vi "Calibration Audit v2.vi"() -> ()   [LabVIEW 2014]
doc: "Obtains calibration information for hardware on selected target."
uses:
  <vilib>/nisyscfg/nisyscfg.lvlib
  <resource>/objmgr/nisysapi.rc
  <vilib>/Utility/miscctls.llb/LVRowAndColumnTypeDef.ctl
  <vilib>/Utility/error.llb/DialogType.ctl
  States.ctl
  <vilib>/Utility/sysdir.llb/System Directory Type.ctl
  <vilib>/Utility/file.llb/Write To Spreadsheet File (string).vi
  <vilib>/nisyscfg/Close (Hardware).vi
  <vilib>/nisyscfg/Close (System).vi
  <vilib>/nisyscfg/Close (Filter).vi
panel:
  in  "Discover Remote Devices?":bool
  in  "Stop Button":bool
  out "Display":string
  in  "User Inputs":T1={"Target "="localhost", "User Name"="", "Password "="", "Filter Enabled?"=FALSE, "Cal File Destination"=path ""}
  in  "START":bool
  out "Calibration Results":string[][](table)
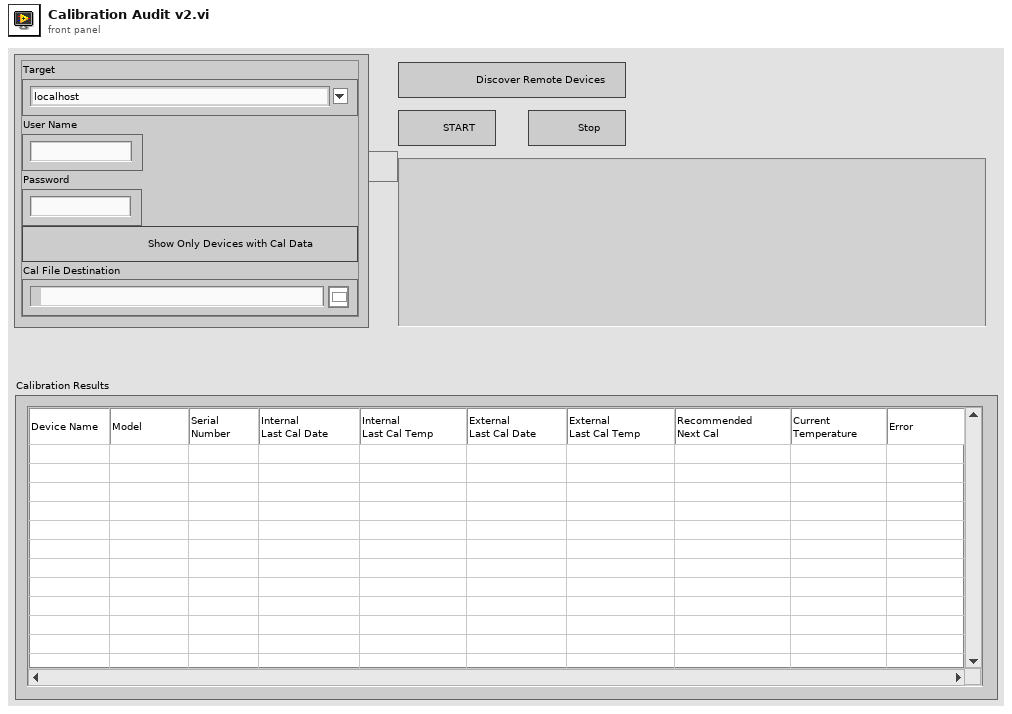
[diagram p1: front panel]
types:
  T1 = cluster{"Target ":string, "User Name":string, "Password ":string, "Filter Enabled?":bool, "Cal File Destination":path}
  T2 = cluster{"SysConfig Session":refnum<k21>, "SysConfig Filter":refnum<k20>, "Modules to Cal":refnum<k20>[], "Cal Data to Write":string[][], "ComboBox Values":string[]}
  T3 = typedef "States.ctl" = enum16{"Initialize", "List Known Systems", "Discover Remote", "Wait for Event", "Filter and Validate", "Update Cal Data", "Report Cal Data", "Close"}
  T4 = cluster{"User Inputs":cluster{"Target ":string, "User Name":string, "Password ":string, "Filter Enabled?":bool, "Cal File Destination":path}, "Display":refnum<vi>, "Target ":refnum<vi>}
  T5 = typedef "LVRowAndColumnTypeDef.ctl" = cluster{"Row":i32, "Column":i32}
  T6 = typedef "System Directory Type.ctl" = i32
  T7 = typedef "DialogType.ctl" = u16
  T8 = cluster{"Last Calibrated":timestamp, "Last Temperature":dbl, "Recommended Next Calibration":timestamp}
  T9 = cluster{"Last Calibrated":timestamp, "Last Temperature":dbl}
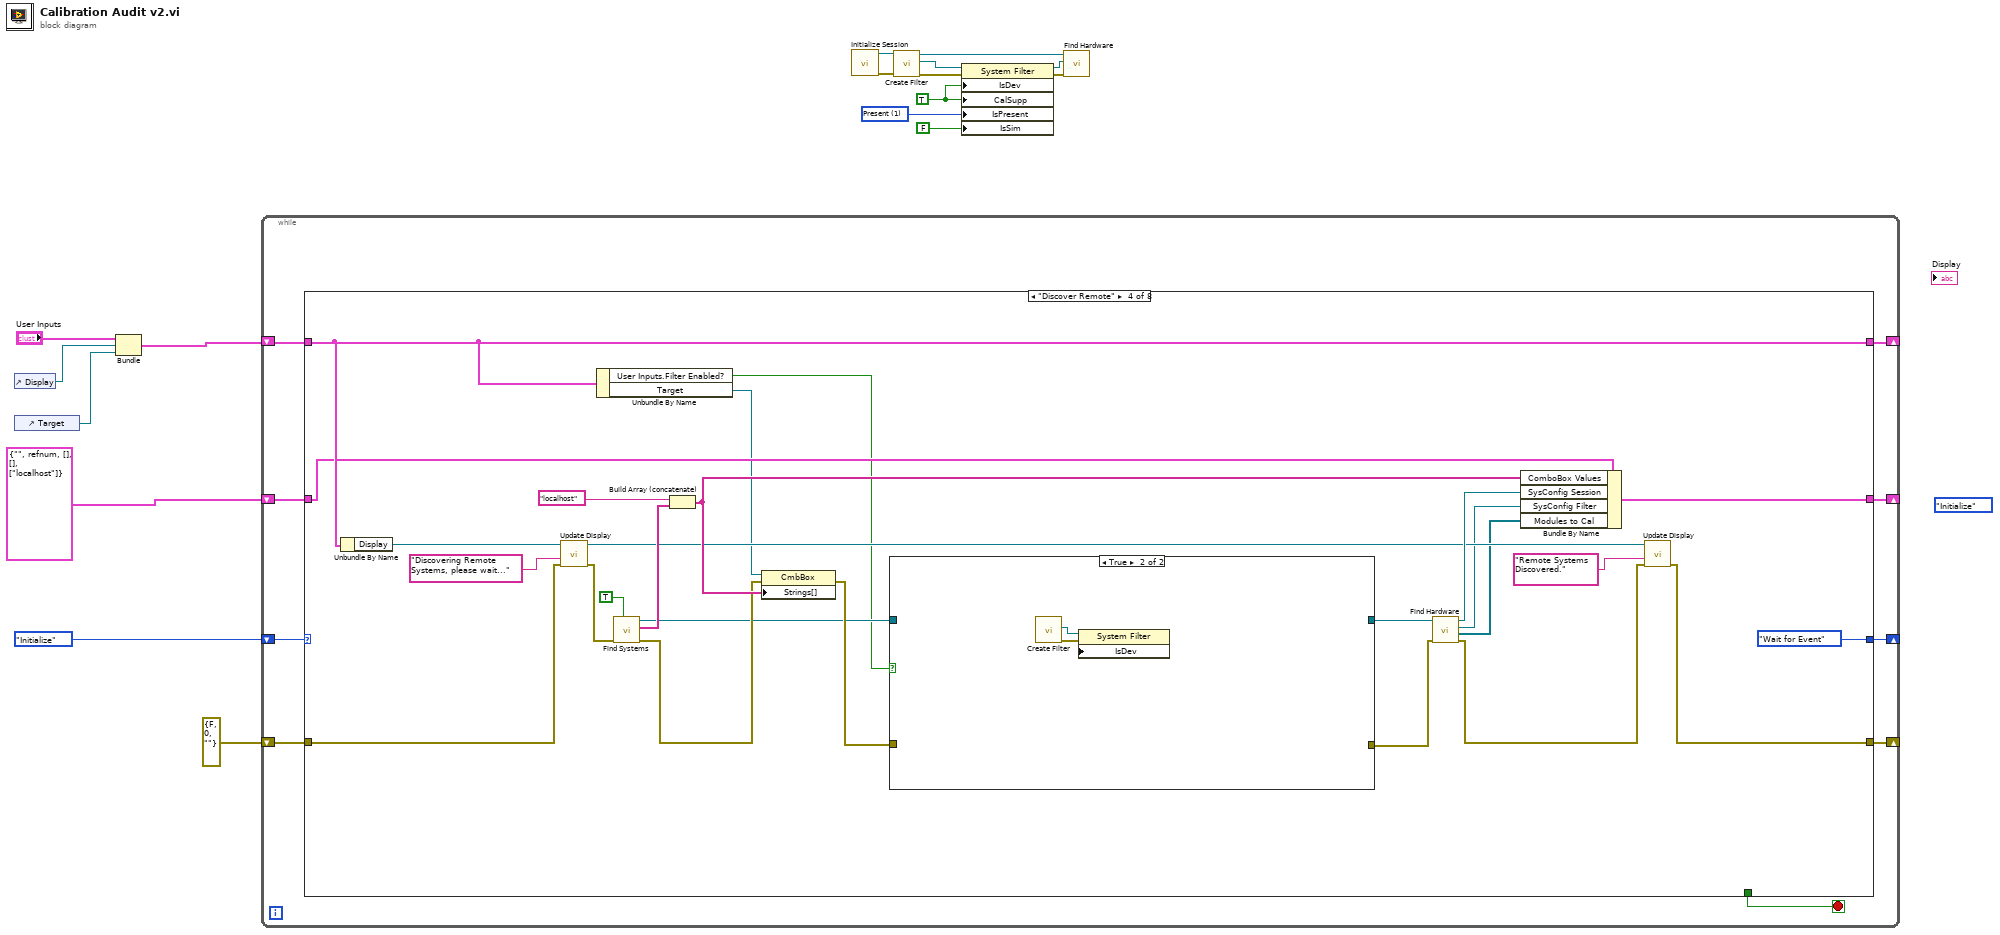
[diagram p0: block diagram]
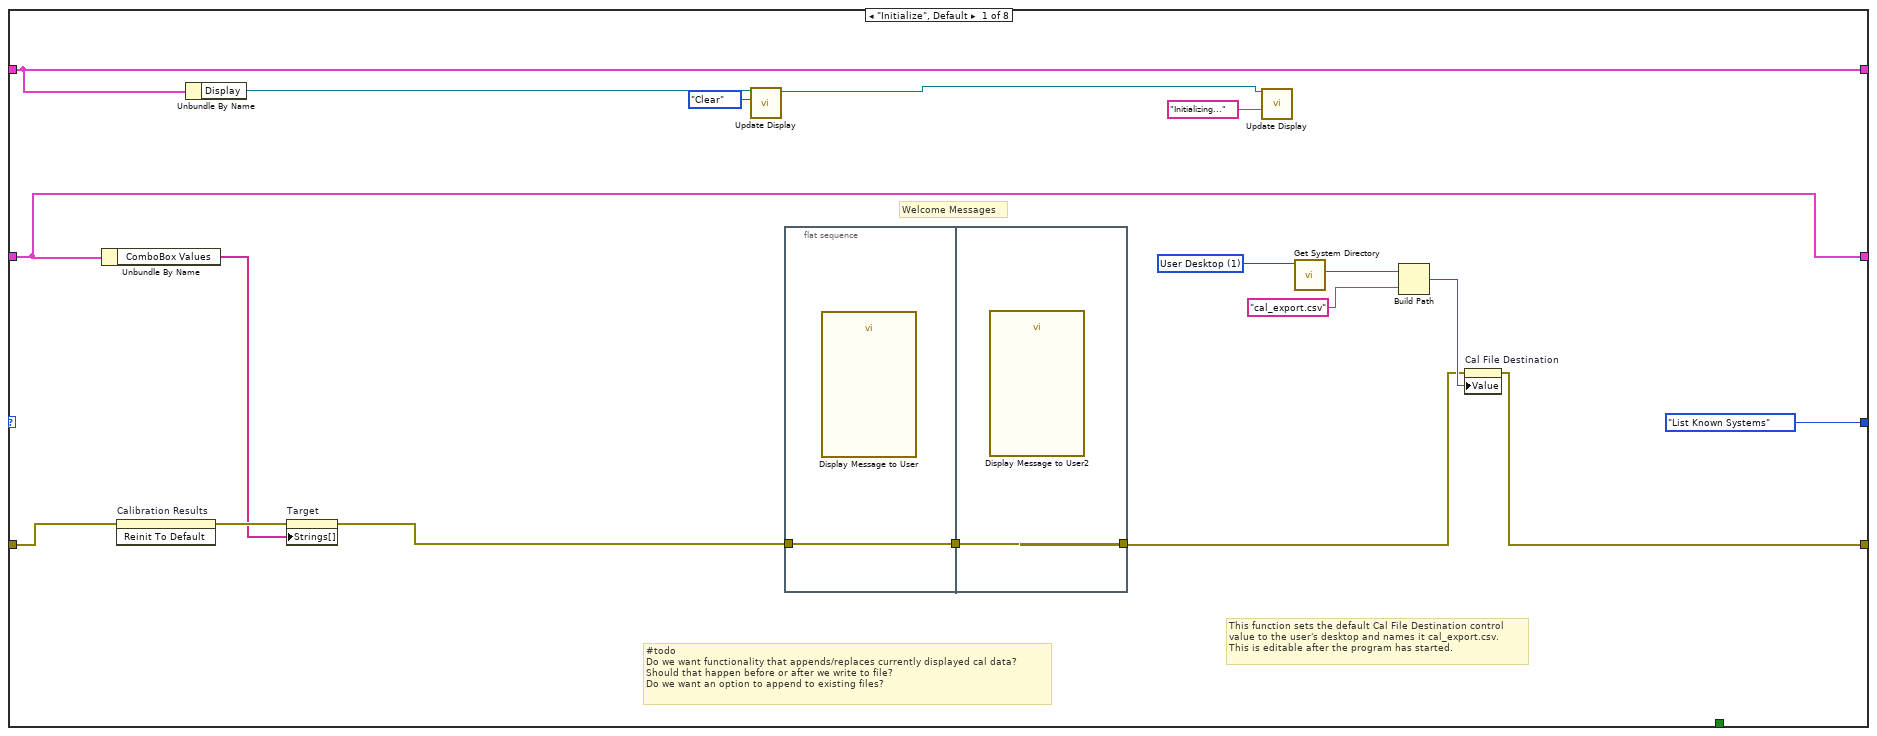
[diagram p2: hidden frame]
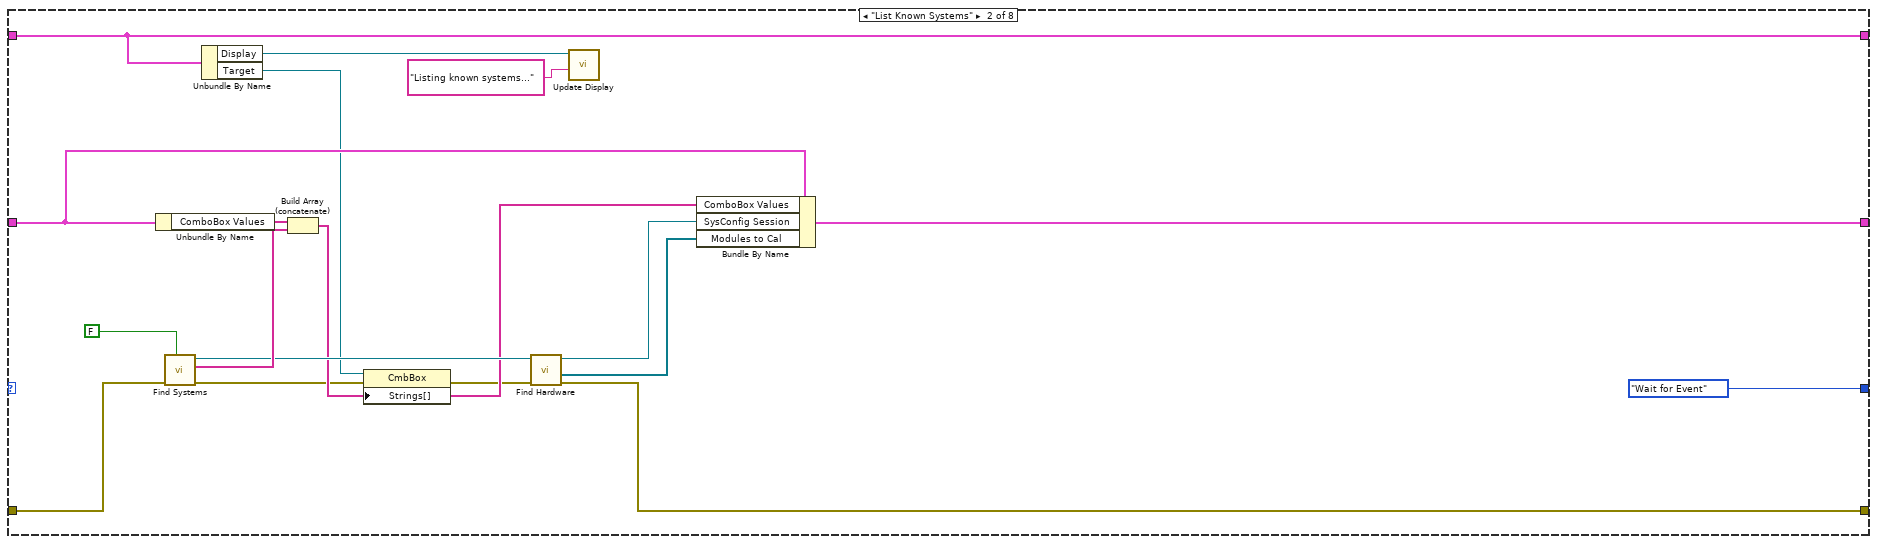
[diagram p3: hidden frame]
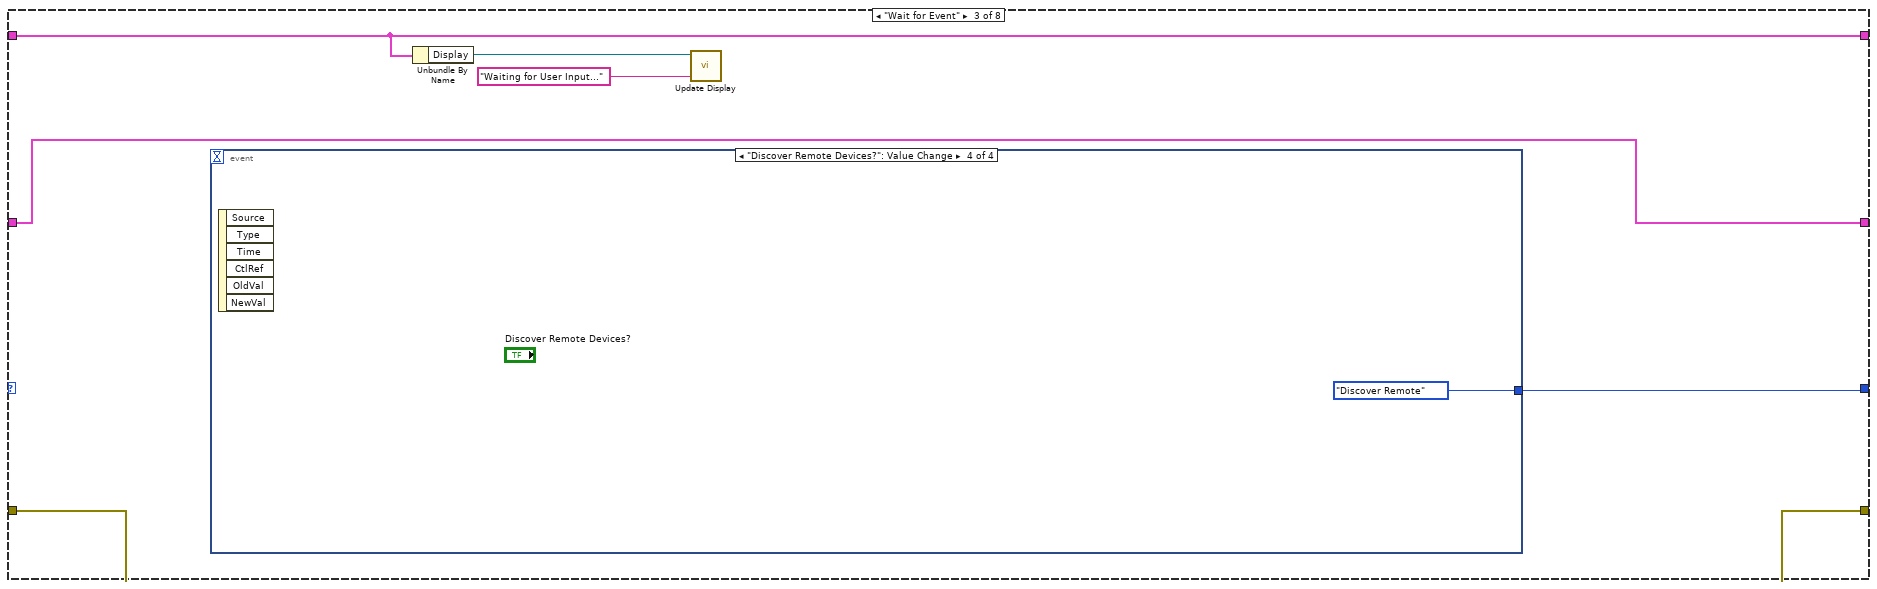
[diagram p4: hidden frame]
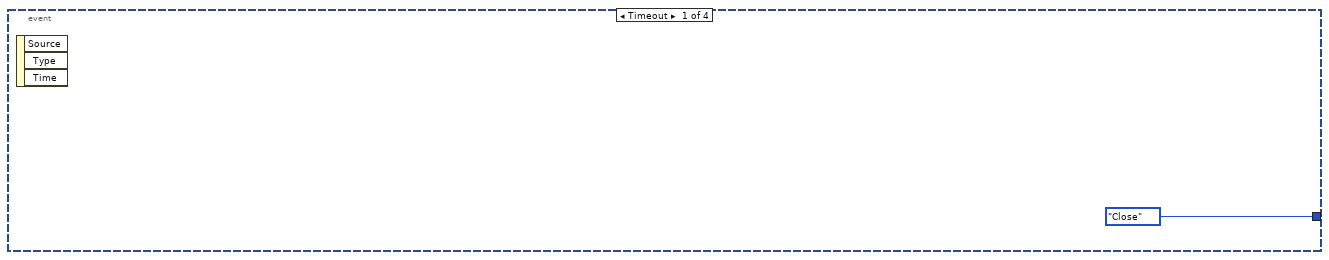
[diagram p5: hidden frame]
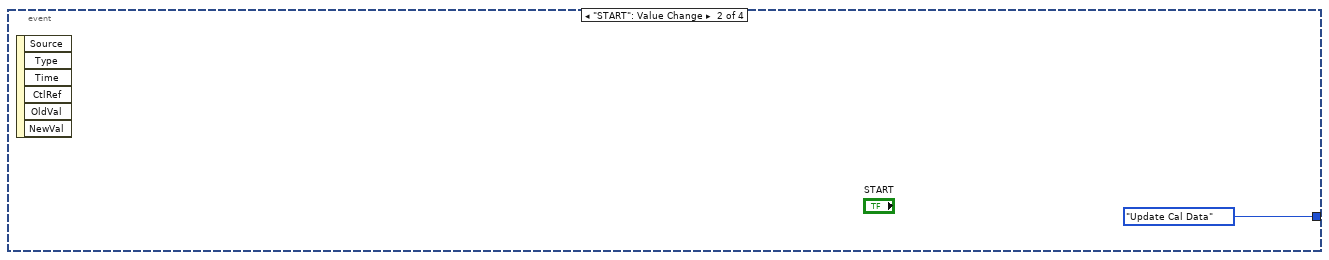
[diagram p6: hidden frame]
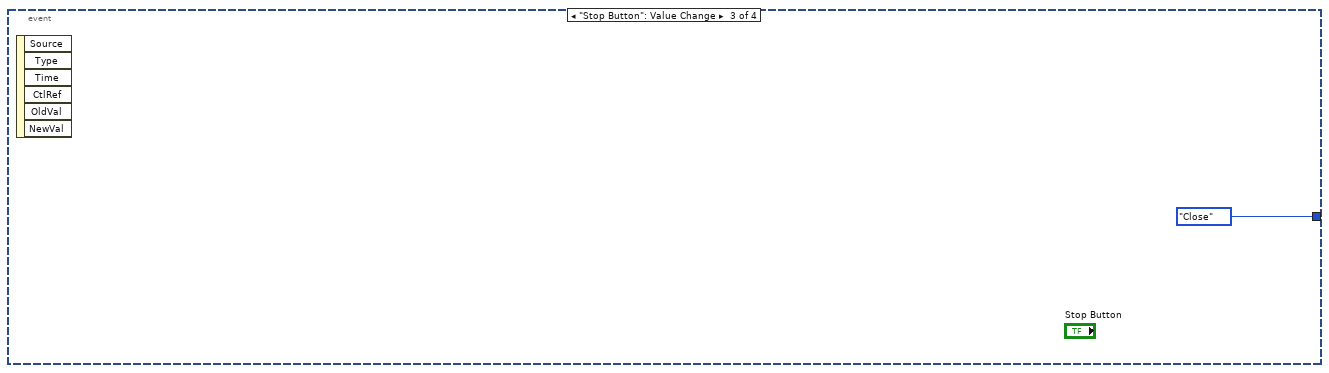
[diagram p7: hidden frame]
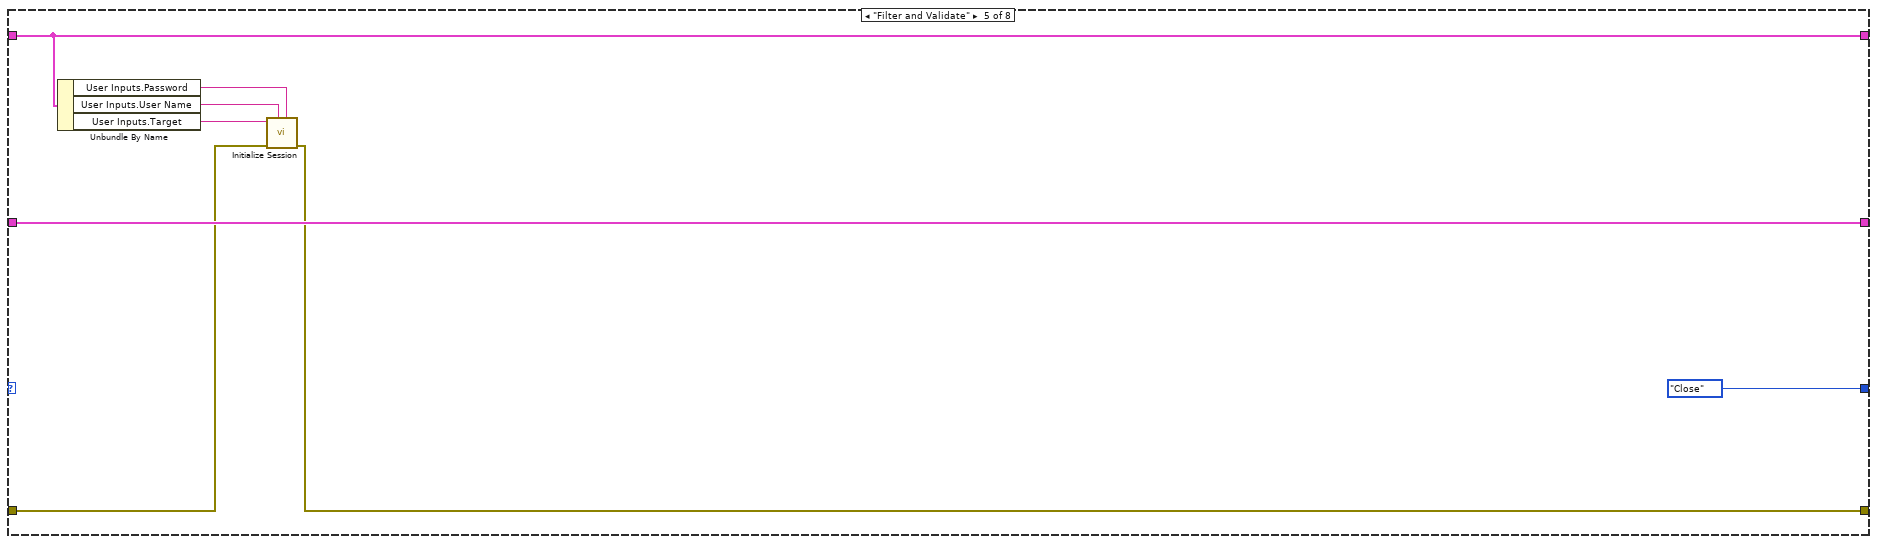
[diagram p9: hidden frame]
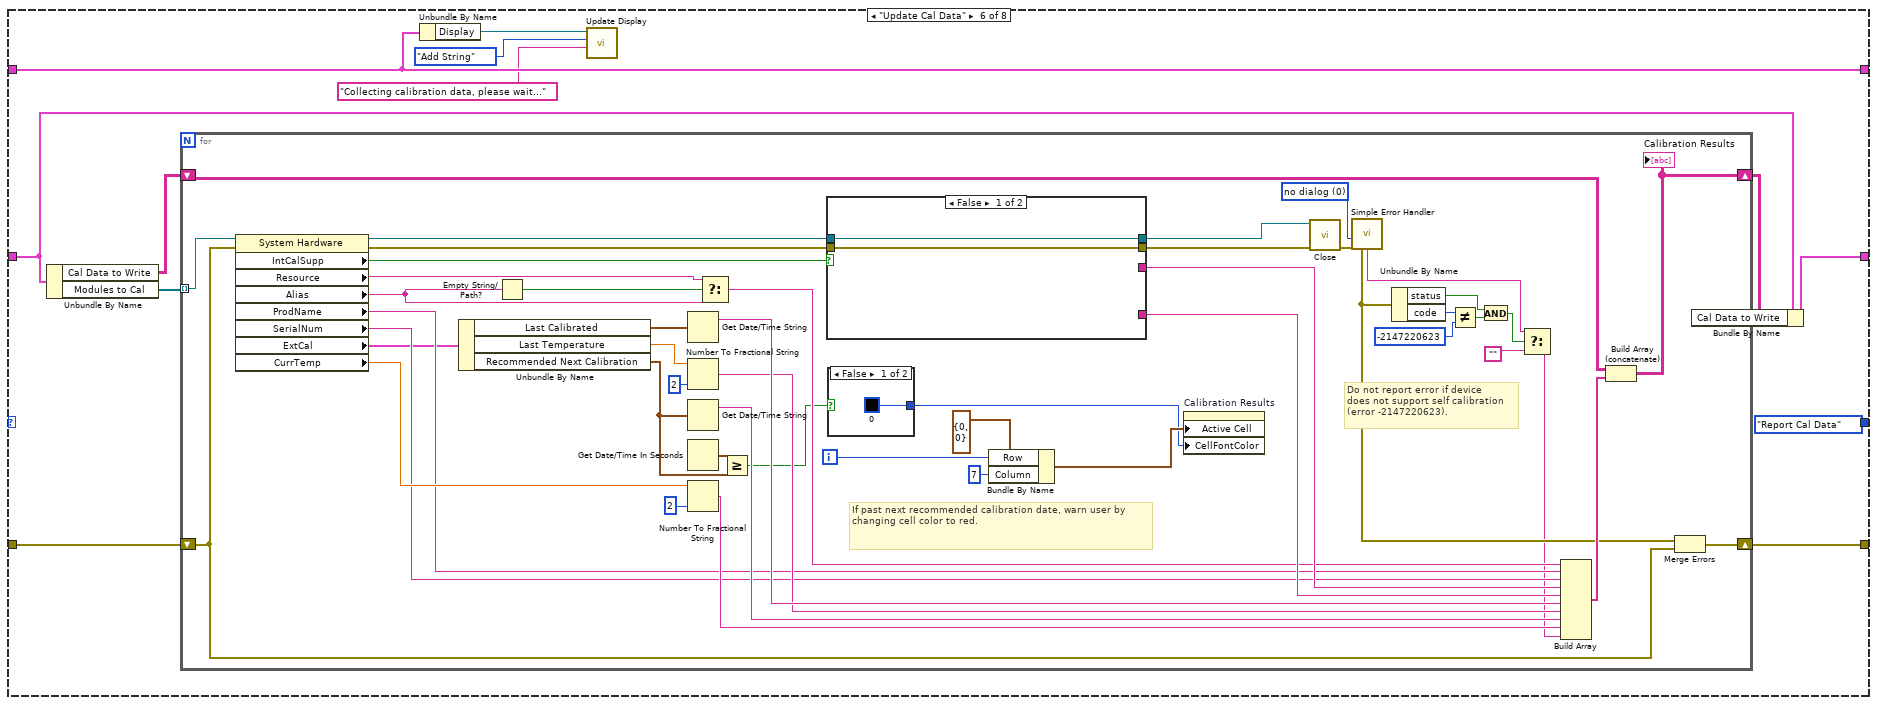
[diagram p10: hidden frame]
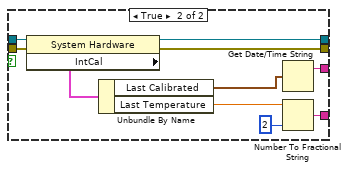
[diagram p11: hidden frame]
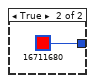
[diagram p12: hidden frame]
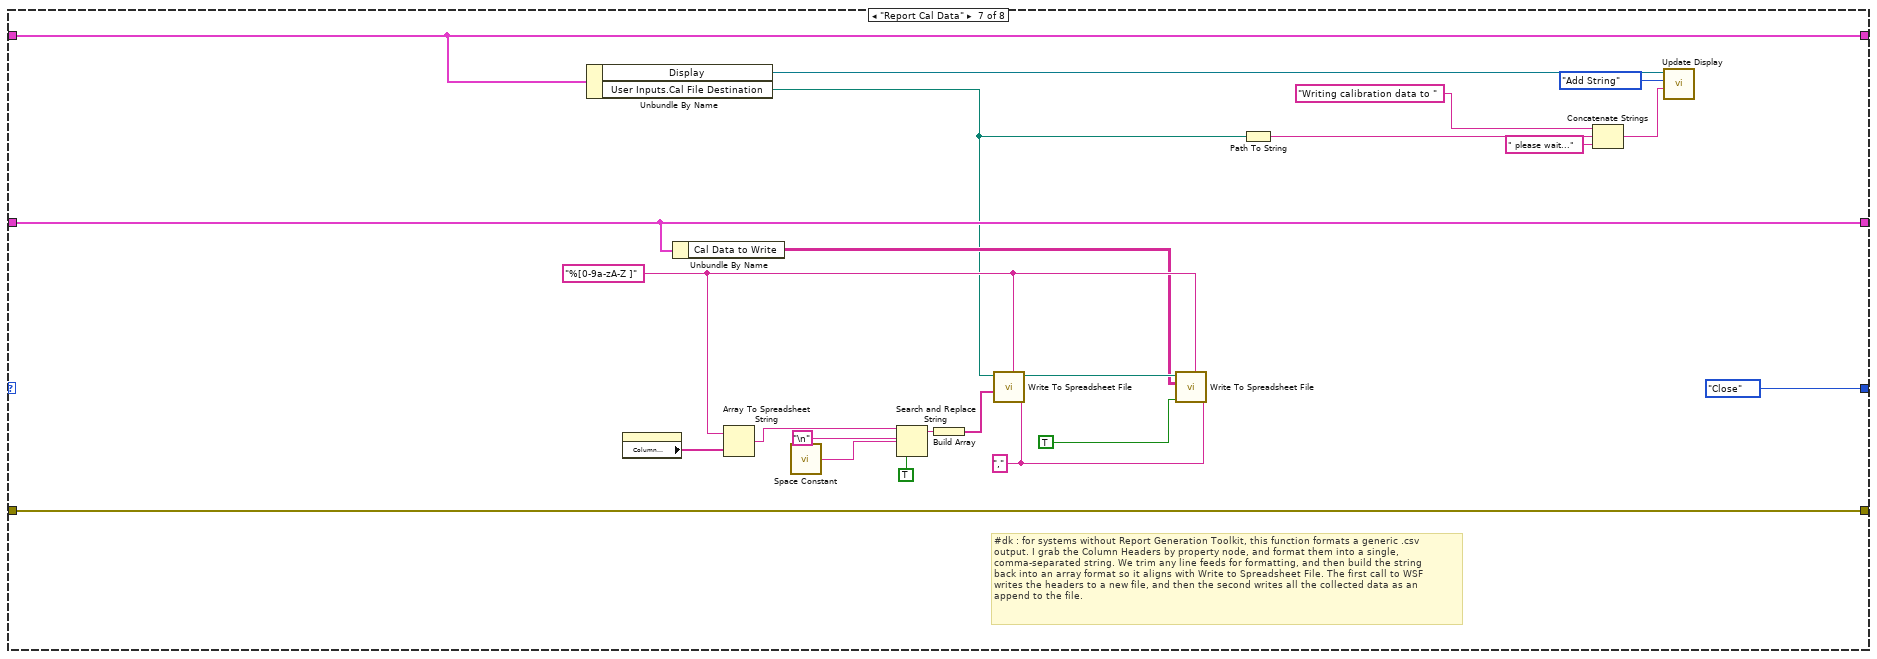
[diagram p13: hidden frame]
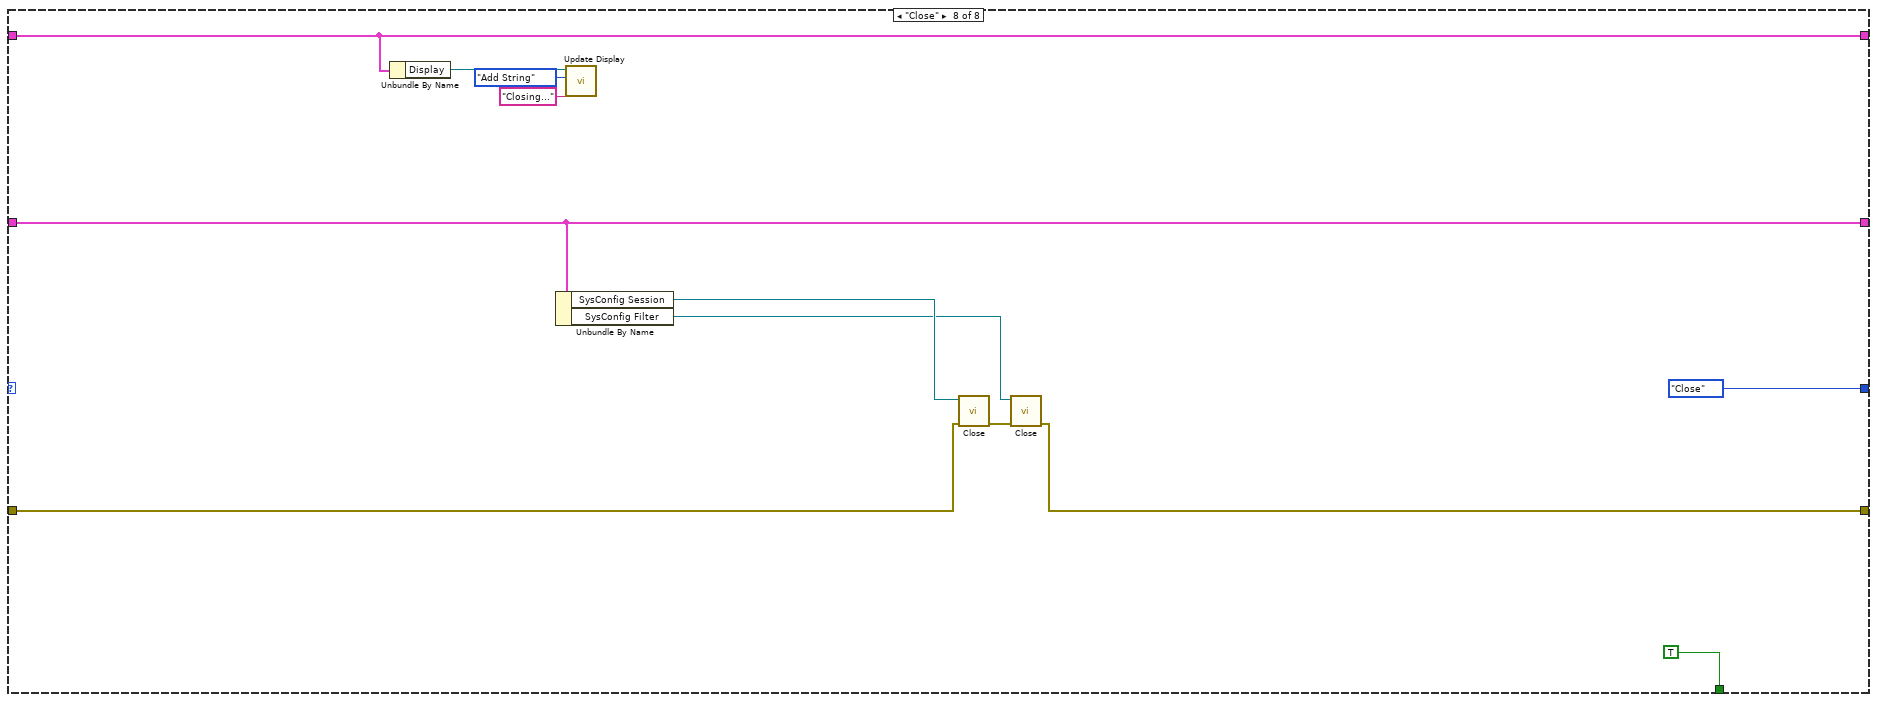
[diagram p14: hidden frame]
diagram:
  (unwired) States."Initialize"
  w13 = 1 items=["Unknown"=-1, "Not Present"=0, "Present"=1] ("Is Present")
  w9 = TRUE ("Is Device")
  n1 = control-ref of="Display"() -> (w2:refnum<vi>)
  n2 = control-ref of="Target"() -> (w1:refnum<vi>)
  n3 = Bundle("User Inputs"="User Inputs", "Display"=w2, "Target"=w1) -> (w5:T4)  [unwired: 1 in]
  n4 = while {
    shift-right: [w22] -> _
    shift-left: States."Initialize" -> [w18]
    shift-right: [w23] -> _
    shift-left: errorcluster {"status"=FALSE, "code"=0, "source"=""} ("error constant") -> [w26]
    shift-right: [w24] -> _
    shift-left: w5 -> [w25]
    shift-right: [w20] -> _
    shift-left: T2 {"SysConfig Session"="", "SysConfig Filter"=refnum, "Modules to Cal"=[], "Cal Data to Write"=[], "ComboBox Values"=["localhost"]} -> [w19]
    stop <- w21 stop-if-true
    n5 = case shown="\"Discover Remote\"" w18 {
      tunnel: w26 -> [w32 w57 w70 w90 w107 w123 w197 w215]
      tunnel: w25 -> [w36 w62 w67 w92 w111 w116 w195 w212]
      tunnel: [w36 w62 w67 w92 w111 w116 w195 w212] -> w24
      tunnel: [w38 w54 w70 w86 w105 w122 w197 w214] -> w23
      tunnel: [States."List Known Systems" States."Wait for Event" w69 States."Wait for Event" States."Close" States."Report Cal Data" States."Close" States."Close"] -> w22
      tunnel: [_ _ _ _ _ _ _ TRUE] -> w21
      tunnel: [w29 w63 w68 w89 w112 w117 w194 w217] -> w20
      tunnel: w19 -> [w29 w59 w68 w84 w112 w118 w194 w217]
      frame "Initialize", Default {
        w44 = T6 1 items=["User Home"=0, "User Desktop"=1, "User Documents"=2, "User Application Data"=3, "User Preferences"=4, "User Temporary"=5, "Public Documents"=6, "Public Application Data"=7, "Public Preferences"=8, "Public Cache"=13, "System Core Libraries"=9, "System Installed Libraries"=10, "Application Files"=11, "Boot Volume Root"=12] ("system directory type")
        # "#todo \nDo we want functionality that appends/replaces currently displayed cal data?\nShould that happen before or after we write to file? \nDo we want an option to append to existing files?"
        # "Welcome Messages"
        # "This function sets the default Cal File Destination control\nvalue to the user's desktop and names it cal_export.csv. \nThis is editable after the program has started."
        n6 = Unbundle By Name(w29) -> ("ComboBox Values"=w28:string[])
        n7 = invoke on="Calibration Results" class="Tbl (strict)" method="Reinit To Default"(error in=w32) -> (error out=w31:errorcluster)  [unwired: 2 in, 2 out]
        n8 = Unbundle By Name(w36) -> ("Display"=w35:refnum<vi>)
        n9 = property on="Target" class="CmbBox"(error in=w31, "Strings[]"=w28) -> (error out=w30:errorcluster)  [unwired: 1 in, 1 out]
        n10 = call "Update Display.vi"("Action"=enum16{"Add String", "Newline", "Clear"}."Clear", "Display In"=w35) -> ("Display Out"=w34:refnum<vi>)  [unwired: 8 in, 1 out]
        n11 = flat-sequence {
          tunnel: w30 -> [w45]
          tunnel: [w45] -> w41
          tunnel: [w46] -> w39
          tunnel: w41 -> [w46]
          frame #0 {
            n12 = call "Display Message to User"() -> ()  [unwired: 10 in, 2 out]
          }
          frame #1 {
            n13 = call "Display Message to User2"() -> ()  [unwired: 10 in, 2 out]
          }
        }
        n14 = call "Update Display.vi"("string"="Initializing...", "Display In"=w34) -> ()  [unwired: 8 in, 2 out]
        n15 = call <vilib>:"Get System Directory.vi"("system directory type"=w44) -> ("system directory"=w42:path)  [unwired: 10 in]
        n16 = Build Path(base path=w42, name or relative path="cal_export.csv") -> (appended path=w40:path)
        n17 = property on="Cal File Destination" class="Path"(error in=w39, "Value"=w40) -> (error out=w38:errorcluster)  [unwired: 1 in, 1 out]
      }
      frame "List Known Systems" {
        n18 = Unbundle By Name(w59) -> ("ComboBox Values"=w56:string[])
        n19 = call <vilib>:"Find Systems.vi"("Detect Online Systems (T)"=FALSE, "error in (no error)"=w57) -> ("error out"=w49:errorcluster, "Detected Systems"=w58:string[], "Session out"=w55:refnum<k21>)  [unwired: 7 in]
        n20 = Unbundle By Name(w62) -> ("Display"=w61:refnum<vi>, "Target"=w51:refnum<vi>)
        n21 = Build Array (concatenate)(w56, w58) -> (w50:string[])
        n22 = property class="CmbBox"(reference=w51, error in=w49, "Strings[]"=w50) -> (error out=w48:errorcluster)  [unwired: 1 out]
        n23 = call <vilib>:"Find Hardware.vi"("error in (no error)"=w48, "Session in"=w55) -> ("error out"=w54:errorcluster, "Resources out"=w52:refnum<k20>[], "Session out"=w53:refnum<k21>)  [unwired: 6 in, 1 out]
        n24 = call "Update Display.vi"("string"="Listing known systems...", "Display In"=w61) -> ()  [unwired: 8 in, 2 out]
        n25 = Bundle By Name(cluster=w59, "ComboBox Values"=w50, "SysConfig Session"=w53, "Modules to Cal"=w52) -> (w63:T2)
      }
      frame "Wait for Event" {
        n26 = event shown="[3] \"Discover Remote Devices?\": Value Change" {
          selector: _ -> [_ _ _ _]
          dyn-events: _ -> [_ _ _ _]
          timeout: _ -> [_ _ _ _]
          tunnel: [States."Close" States."Update Cal Data" States."Close" States."Discover Remote"] -> w69
          event Timeout {
            n27 = event-data() -> ()  [unwired: 1 in, 3 out]
          }
          event "START": Value Change {
            n28 = event-data() -> ()  [unwired: 1 in, 6 out]
          }
          event "Stop Button": Value Change {
            n29 = event-data() -> ()  [unwired: 1 in, 6 out]
          }
          event "Discover Remote Devices?": Value Change {
            n30 = event-data() -> ()  [unwired: 1 in, 6 out]
          }
        }
        n31 = Unbundle By Name(w67) -> ("Display"=w66:refnum<vi>)
        n32 = call "Update Display.vi"("string"="Waiting for User Input...", "Display In"=w66) -> ()  [unwired: 8 in, 2 out]
      }
      frame "Discover Remote" {
        n33 = Unbundle By Name(w92) -> ("Display"=w91:refnum<vi>)
        n34 = call "Update Display.vi"("Error In"=w90, "string"="Discovering Remote Systems, please wait...", "Display In"=w91) -> ("Error Out"=w93:errorcluster, "Display Out"=w88:refnum<vi>)  [unwired: 7 in]
        n35 = Unbundle By Name(w92) -> ("User Inputs.Filter Enabled?"=w77:bool, "Target"=w82:refnum<vi>)
        n36 = call <vilib>:"Find Systems.vi"("Detect Online Systems (T)"=TRUE, "error in (no error)"=w93) -> ("error out"=w95:errorcluster, "Detected Systems"=w98:string[], "Session out"=w79:refnum<k21>)  [unwired: 7 in]
        n37 = Build Array (concatenate)("localhost", w98) -> (w96:string[])
        n38 = property class="CmbBox"(reference=w82, error in=w95, "Strings[]"=w96) -> (error out=w81:errorcluster)  [unwired: 1 out]
        n39 = case shown="True" w77 {
          tunnel: w81 -> [w102 _]
          tunnel: [w102 _] -> w80
          tunnel: w79 -> [w101 _]
          tunnel: [w101 _] -> w78
          frame False {
          }
          frame True {
            n40 = call <vilib>:"Create Filter.vi"() -> ("error out"=w104:errorcluster, "Filter out"=w103:refnum<k20>)  [unwired: 9 in, 1 out]
            n41 = property class="System Filter" props=["IsDev"](reference=w103, error in=w104) -> ()  [unwired: 1 in, 2 out]
          }
        }
        n42 = call <vilib>:"Find Hardware.vi"("error in (no error)"=w80, "Session in"=w78) -> ("error out"=w87:errorcluster, "Resources out"=w76:refnum<k20>[], "Filter out"=w75:refnum<k20>, "Session out"=w97:refnum<k21>)  [unwired: 6 in]
        n43 = Bundle By Name(cluster=w84, "ComboBox Values"=w96, "SysConfig Session"=w97, "SysConfig Filter"=w75, "Modules to Cal"=w76) -> (w89:T2)
        n44 = call "Update Display.vi"("Error In"=w87, "string"="Remote Systems Discovered.", "Display In"=w88) -> ("Error Out"=w86:errorcluster)  [unwired: 7 in, 1 out]
      }
      frame "Filter and Validate" {
        n45 = Unbundle By Name(w111) -> ("User Inputs.Password"=w108:string, "User Inputs.User Name"=w109:string, "User Inputs.Target"=w110:string)
        n46 = call <vilib>:"Initialize Session.vi"("Password"=w108, "User Name"=w109, "error in (no error)"=w107, "Target (localhost)"=w110) -> ("error out"=w105:errorcluster)  [unwired: 6 in, 1 out]
      }
      frame "Update Cal Data" {
        n47 = Unbundle By Name(w118) -> ("Cal Data to Write"=w120:string[][], "Modules to Cal"=w121:refnum<k20>[])
        n48 = for {
          shift-right: [w126] -> w119
          shift-left: w120 -> [w170]
          shift-right: [w128] -> w122
          shift-left: w123 -> [w129]
          tunnel: w121 -> [w125] mode=indexing
          i -> [w149]
          w148 = T7 0 items=["no dialog", "OK message", "continue or stop message", "OK message + warnings", "continue/stop + warnings"] ("type of dialog (OK msg:1)")
          # "If past next recommended calibration date, warn user by \nchanging cell color to red."
          # "Do not report error if device \ndoes not support self calibration\n(error -2147220623)."
          n49 = property class="System Hardware"(reference=w125, error in=w129) -> (reference out=w136:refnum<k20>, error out=w143:errorcluster, "IntCalSupp"=w137:bool, "Resource"=w138:string, "Alias"=w139:string, "ProdName"=w157:string, "SerialNum"=w156:string, "ExtCal"=w147:T8, "CurrTemp"=w164:dbl)
          n50 = Unbundle By Name(w147) -> ("Last Calibrated"=w141:timestamp, "Last Temperature"=w166:dbl, "Recommended Next Calibration"=w140:timestamp)
          n51 = Empty String/Path?(string/path=w139) -> (empty?=w171:bool)
          n52 = Get Date/Time String(seconds (now)=w141) -> (date string=w161:string)  [unwired: 2 in, 1 out]
          n53 = Number To Fractional String(number=w166, precision (6)=i16 2) -> (F-format string=w160:string)  [unwired: 2 in]
          n54 = Get Date/Time String(seconds (now)=w140) -> (date string=w159:string)  [unwired: 2 in, 1 out]
          n55 = Get Date/Time In Seconds() -> (seconds since 1Jan1904=w150:timestamp)
          n56 = Number To Fractional String(number=w164, precision (6)=i16 2) -> (F-format string=w163:string)  [unwired: 2 in]
          n57 = Select(t=w138, s=w171, f=w139) -> (s? t:f=w158:string)
          n58 = Greater Or Equal?(x=w150, y=w140) -> (x >= y?=w152:bool)
          n59 = case shown="False" w137 {
            tunnel: [_ w183] -> w168
            tunnel: [_ w182] -> w167
            tunnel: [w172 w178] -> w144
            tunnel: w143 -> [w173 w177]
            tunnel: [w173 w176] -> w142
            tunnel: w136 -> [w172 w174]
            frame False {
            }
            frame True {
              n60 = property class="System Hardware"(reference=w174, error in=w177) -> (reference out=w178:refnum<k20>, error out=w176:errorcluster, "IntCal"=w175:T9)
              n61 = Unbundle By Name(w175) -> ("Last Calibrated"=w180:timestamp, "Last Temperature"=w179:dbl)
              n62 = Get Date/Time String(seconds (now)=w180) -> (date string=w183:string)  [unwired: 2 in, 1 out]
              n63 = Number To Fractional String(number=w179, precision (6)=i16 2) -> (F-format string=w182:string)  [unwired: 2 in]
            }
          }
          n64 = case shown="False" w152 {
            tunnel: [u32 0 u32 16711680] -> w153
            frame False {
            }
            frame True {
            }
          }
          n65 = Bundle By Name(cluster=T5 {"Row"=0, "Column"=0} ("Active Cell:Active Cell"), "Row"=w149, "Column"=7) -> (w154:T5)
          n66 = property on="Calibration Results" class="Tbl (strict)"("Active Cell"=w154, "CellFontColor"=w153) -> ()  [unwired: 2 in, 2 out]
          n67 = call-poly <vilib>:"Close.vi"("error in (no error)"=w142, "Resource in"=w144) -> ("error out"=w130:errorcluster)  [unwired: 9 in]
          n68 = call <vilib>:"Simple Error Handler.vi"("type of dialog (OK msg:1)"=w148, "error in (no error)"=w130) -> ("message"=w146:string)  [unwired: 3 in, 4 out]
          n69 = Unbundle By Name(w130) -> ("status"=w134:bool, "code"=w132:i32)
          n70 = Not Equal?(x=w132, y=-2147220623) -> (x != y?=w133:bool)
          n71 = And(x=w134, y=w133) -> (x .and. y?=w135:bool)
          n72 = Select(t=w146, s=w135, f="") -> (s? t:f=w127:string)
          n73 = Build Array(w158, w157, w156, w168, w167, w161, w160, w159, w163, w127) -> (w169:string[])
          n74 = Build Array (concatenate)(w170, w169) -> (w126:string[][])
          "Calibration Results" <- w126
          n75 = Merge Errors(w130, w129) -> (w128:errorcluster)
        }
        n76 = Unbundle By Name(w116) -> ("Display"=w115:refnum<vi>)
        n77 = call "Update Display.vi"("string"="Collecting calibration data, please wait...", "Action"=enum16{"Add String", "Newline", "Clear"}."Add String", "Display In"=w115) -> ()  [unwired: 7 in, 2 out]
        n78 = Bundle By Name(cluster=w118, "Cal Data to Write"=w119) -> (w117:T2)
      }
      frame "Report Cal Data" {
        w205 = "%[0-9a-zA-Z ]" ("format (%s)")
        w204 = "," ("delimiter (\\t)")
        # "#dk : for systems without Report Generation Toolkit, this function formats a generic .csv\noutput. I grab the Column Headers by property node, and format them into a single,\ncomma-separated string. We trim any line feeds for formatting, and then build the string\nback into an array format so it aligns with Write to Spreadsheet File. The first call to WSF\nwrites the headers to a new file, and then the second writes all the collected data as an \nappend to the file."
        n79 = Unbundle By Name(w195) -> ("Display"=w192:refnum<vi>, "User Inputs.Cal File Destination"=w189:path)
        n80 = property on="Calibration Results" class="Tbl (strict)"() -> ("Column Headers[]"=w206:string[])  [unwired: 2 in, 2 out]
        n81 = Unbundle By Name(w194) -> ("Cal Data to Write"=w193:string[][])
        n82 = Array To Spreadsheet String(array=w206, 3:w205) -> (spreadsheet string=w202:string)  [unwired: 1 in]
        n83 = call <vilib>:"Space Constant.vi"() -> ("String"=w199:string)
        n84 = Search and Replace String(replace all?=TRUE ("replace all? (F)"), input string=w202, search string="\n", replace string=w199) -> (result string=w203:string)  [unwired: 4 in, 3 out]
        n85 = Build Array(w203) -> (w198:string[])
        n86 = call-poly <vilib>:"Write To Spreadsheet File.vi"("delimiter (\\t)"=w204, "format (%s)"=w205, "1D data"=w198, "file path (dialog if empty)"=w189) -> ("new file path (Not A Path if cancelled)"=w208:path)  [unwired: 4 in]
        n87 = call-poly <vilib>:"Write To Spreadsheet File.vi"("delimiter (\\t)"=w204, "format (%s)"=w205, "append to file? (new file:F)"=TRUE, "2D data"=w193, "file path (dialog if empty)"=w208) -> ()  [unwired: 3 in, 1 out]
        n88 = Path To String(path=w189) -> (string=w190:string)
        n89 = Concatenate Strings("Writing calibration data to " ("string"), w190, " please wait..." ("string")) -> (w186:string)
        n90 = call "Update Display.vi"("string"=w186, "Action"=enum16{"Add String", "Newline", "Clear"}."Add String", "Display In"=w192) -> ()  [unwired: 7 in, 2 out]
      }
      frame "Close" {
        n91 = Unbundle By Name(w212) -> ("Display"=w211:refnum<vi>)
        n92 = Unbundle By Name(w217) -> ("SysConfig Session"=w216:refnum<k21>, "SysConfig Filter"=w213:refnum<k20>)
        n93 = call "Update Display.vi"("string"="Closing...", "Action"=enum16{"Add String", "Newline", "Clear"}."Add String", "Display In"=w211) -> ()  [unwired: 7 in, 2 out]
        n94 = call-poly <vilib>:"Close.vi"("error in (no error)"=w215, "Session in"=w216) -> ("error out"=w220:errorcluster)  [unwired: 9 in]
        n95 = call-poly <vilib>:"Close.vi"("error in (no error)"=w220, "Filter in"=w213) -> ("error out"=w214:errorcluster)  [unwired: 9 in]
      }
    }
  }
  n96 = call <vilib>:"Initialize Session.vi"() -> ("error out"=w15:errorcluster, "Session out"=w16:refnum<k21>)  [unwired: 10 in]
  n97 = call <vilib>:"Create Filter.vi"("error in (no error)"=w15, "Session in"=w16) -> ("error out"=w8:errorcluster, "Filter out"=w7:refnum<k20>, "Session out"=w12:refnum<k21>)  [unwired: 7 in]
  n98 = property class="System Filter"(reference=w7, error in=w8, "IsDev"=w9, "CalSupp"=w9, "IsPresent"=w13, "IsSim"=FALSE ("Is Simulated")) -> (reference out=w11:refnum<k20>, error out=w10:errorcluster)
  n99 = call <vilib>:"Find Hardware.vi"("error in (no error)"=w10, "Filter in"=w11, "Session in"=w12) -> ()  [unwired: 1 in, 8 out]
